vi "cam4 analyse.vi"() -> (0 "O8 chiffre":string, 1 "O7 chiffre":string, 2 "O1 chiffre":string, 3 "O2 chiffre":string, 4 "O5 chiffre":string, 5 "Y3 chiffre":string, 6 "Y6 chiffre":string, 7 "Y7 chiffre":string)   [LabVIEW 2019]
uses:
  <vilib>/vision/Classification.llb/IMAQ Classifier Read Options.ctl
  <vilib>/vision/NI_Vision_Development_Module.lvlib
panel:
  out "Coordinates":i32[](array[numeric])
  in  "Y7":T1={"Global Rectangle"=[0, 0, 1279, 959], "Contours"=[{"ID"=enum."External", "Type"=3, "Coordinates"=[0, 0, 1279, 959]}]} {"Contours"."Type" items=["No Selection", "Point", "Line", "Rectangle", "Oval", "Polygon", "Freehand Region", "Annulus", "Unused2", "Unused3", "Broken Line", "Freehand Line", "Rotated Rectangle"]}
  out "Y7":string[](array[string])
  in  "Y6":T1={"Global Rectangle"=[0, 0, 1279, 959], "Contours"=[{"ID"=enum."External", "Type"=3, "Coordinates"=[0, 0, 1279, 959]}]} {"Contours"."Type" items=["No Selection", "Point", "Line", "Rectangle", "Oval", "Polygon", "Freehand Region", "Annulus", "Unused2", "Unused3", "Broken Line", "Freehand Line", "Rotated Rectangle"]}
  out "Y6":string[](array[string])
  in  "Y3":T1={"Global Rectangle"=[0, 0, 1279, 959], "Contours"=[{"ID"=enum."External", "Type"=3, "Coordinates"=[0, 0, 1279, 959]}]} {"Contours"."Type" items=["No Selection", "Point", "Line", "Rectangle", "Oval", "Polygon", "Freehand Region", "Annulus", "Unused2", "Unused3", "Broken Line", "Freehand Line", "Rotated Rectangle"]}
  out "Y3":string[](array[string])
  in  "O1":T1={"Global Rectangle"=[0, 0, 1279, 959], "Contours"=[{"ID"=enum."External", "Type"=3, "Coordinates"=[0, 0, 1279, 959]}]} {"Contours"."Type" items=["No Selection", "Point", "Line", "Rectangle", "Oval", "Polygon", "Freehand Region", "Annulus", "Unused2", "Unused3", "Broken Line", "Freehand Line", "Rotated Rectangle"]}
  out "O1":string[](array[string])
  in  "O2":T1={"Global Rectangle"=[0, 0, 1279, 959], "Contours"=[{"ID"=enum."External", "Type"=3, "Coordinates"=[0, 0, 1279, 959]}]} {"Contours"."Type" items=["No Selection", "Point", "Line", "Rectangle", "Oval", "Polygon", "Freehand Region", "Annulus", "Unused2", "Unused3", "Broken Line", "Freehand Line", "Rotated Rectangle"]}
  out "O2":string[](array[string])
  in  "O5":T1={"Global Rectangle"=[0, 0, 1279, 959], "Contours"=[{"ID"=enum."External", "Type"=3, "Coordinates"=[0, 0, 1279, 959]}]} {"Contours"."Type" items=["No Selection", "Point", "Line", "Rectangle", "Oval", "Polygon", "Freehand Region", "Annulus", "Unused2", "Unused3", "Broken Line", "Freehand Line", "Rotated Rectangle"]}
  out "O5":string[](array[string])
  in  "O7":T1={"Global Rectangle"=[0, 0, 1279, 959], "Contours"=[{"ID"=enum."External", "Type"=3, "Coordinates"=[0, 0, 1279, 959]}]} {"Contours"."Type" items=["No Selection", "Point", "Line", "Rectangle", "Oval", "Polygon", "Freehand Region", "Annulus", "Unused2", "Unused3", "Broken Line", "Freehand Line", "Rotated Rectangle"]}
  out "O7":string[](array[string])
  in  "O8":T1={"Global Rectangle"=[640, 450, 686, 504], "Contours"=[{"ID"=enum."External", "Type"=3, "Coordinates"=[640, 450, 686, 504]}]} {"Contours"."Type" items=["No Selection", "Point", "Line", "Rectangle", "Oval", "Polygon", "Freehand Region", "Annulus", "Unused2", "Unused3", "Broken Line", "Freehand Line", "Rotated Rectangle"]}
  out "Image Out 2":T2(plugin-control)
  out "error out 2":errorcluster
  out "O8":string[](array[string])
  in  "error in":errorcluster
types:
  T1 = cluster{"Global Rectangle":i32[], "Contours":cluster{"ID":enum32{"External", "Internal"}, "Type":u32, "Coordinates":i32[]}[]}
  T2 = typedef "IMAQ Image.ctl" = refnum<image>
  T3 = typedef "IMAQ Classifier Read Options.ctl" = i32
  T4 = typedef "IMAQ Classifier Session.ctl" = refnum<k1>
  T5 = typedef "ROI Descriptor" = cluster{"Global Rectangle":i32[], "Contours":cluster{"ID":enum32{"External", "Internal"}, "Type":u32, "Coordinates":i32[]}[]}
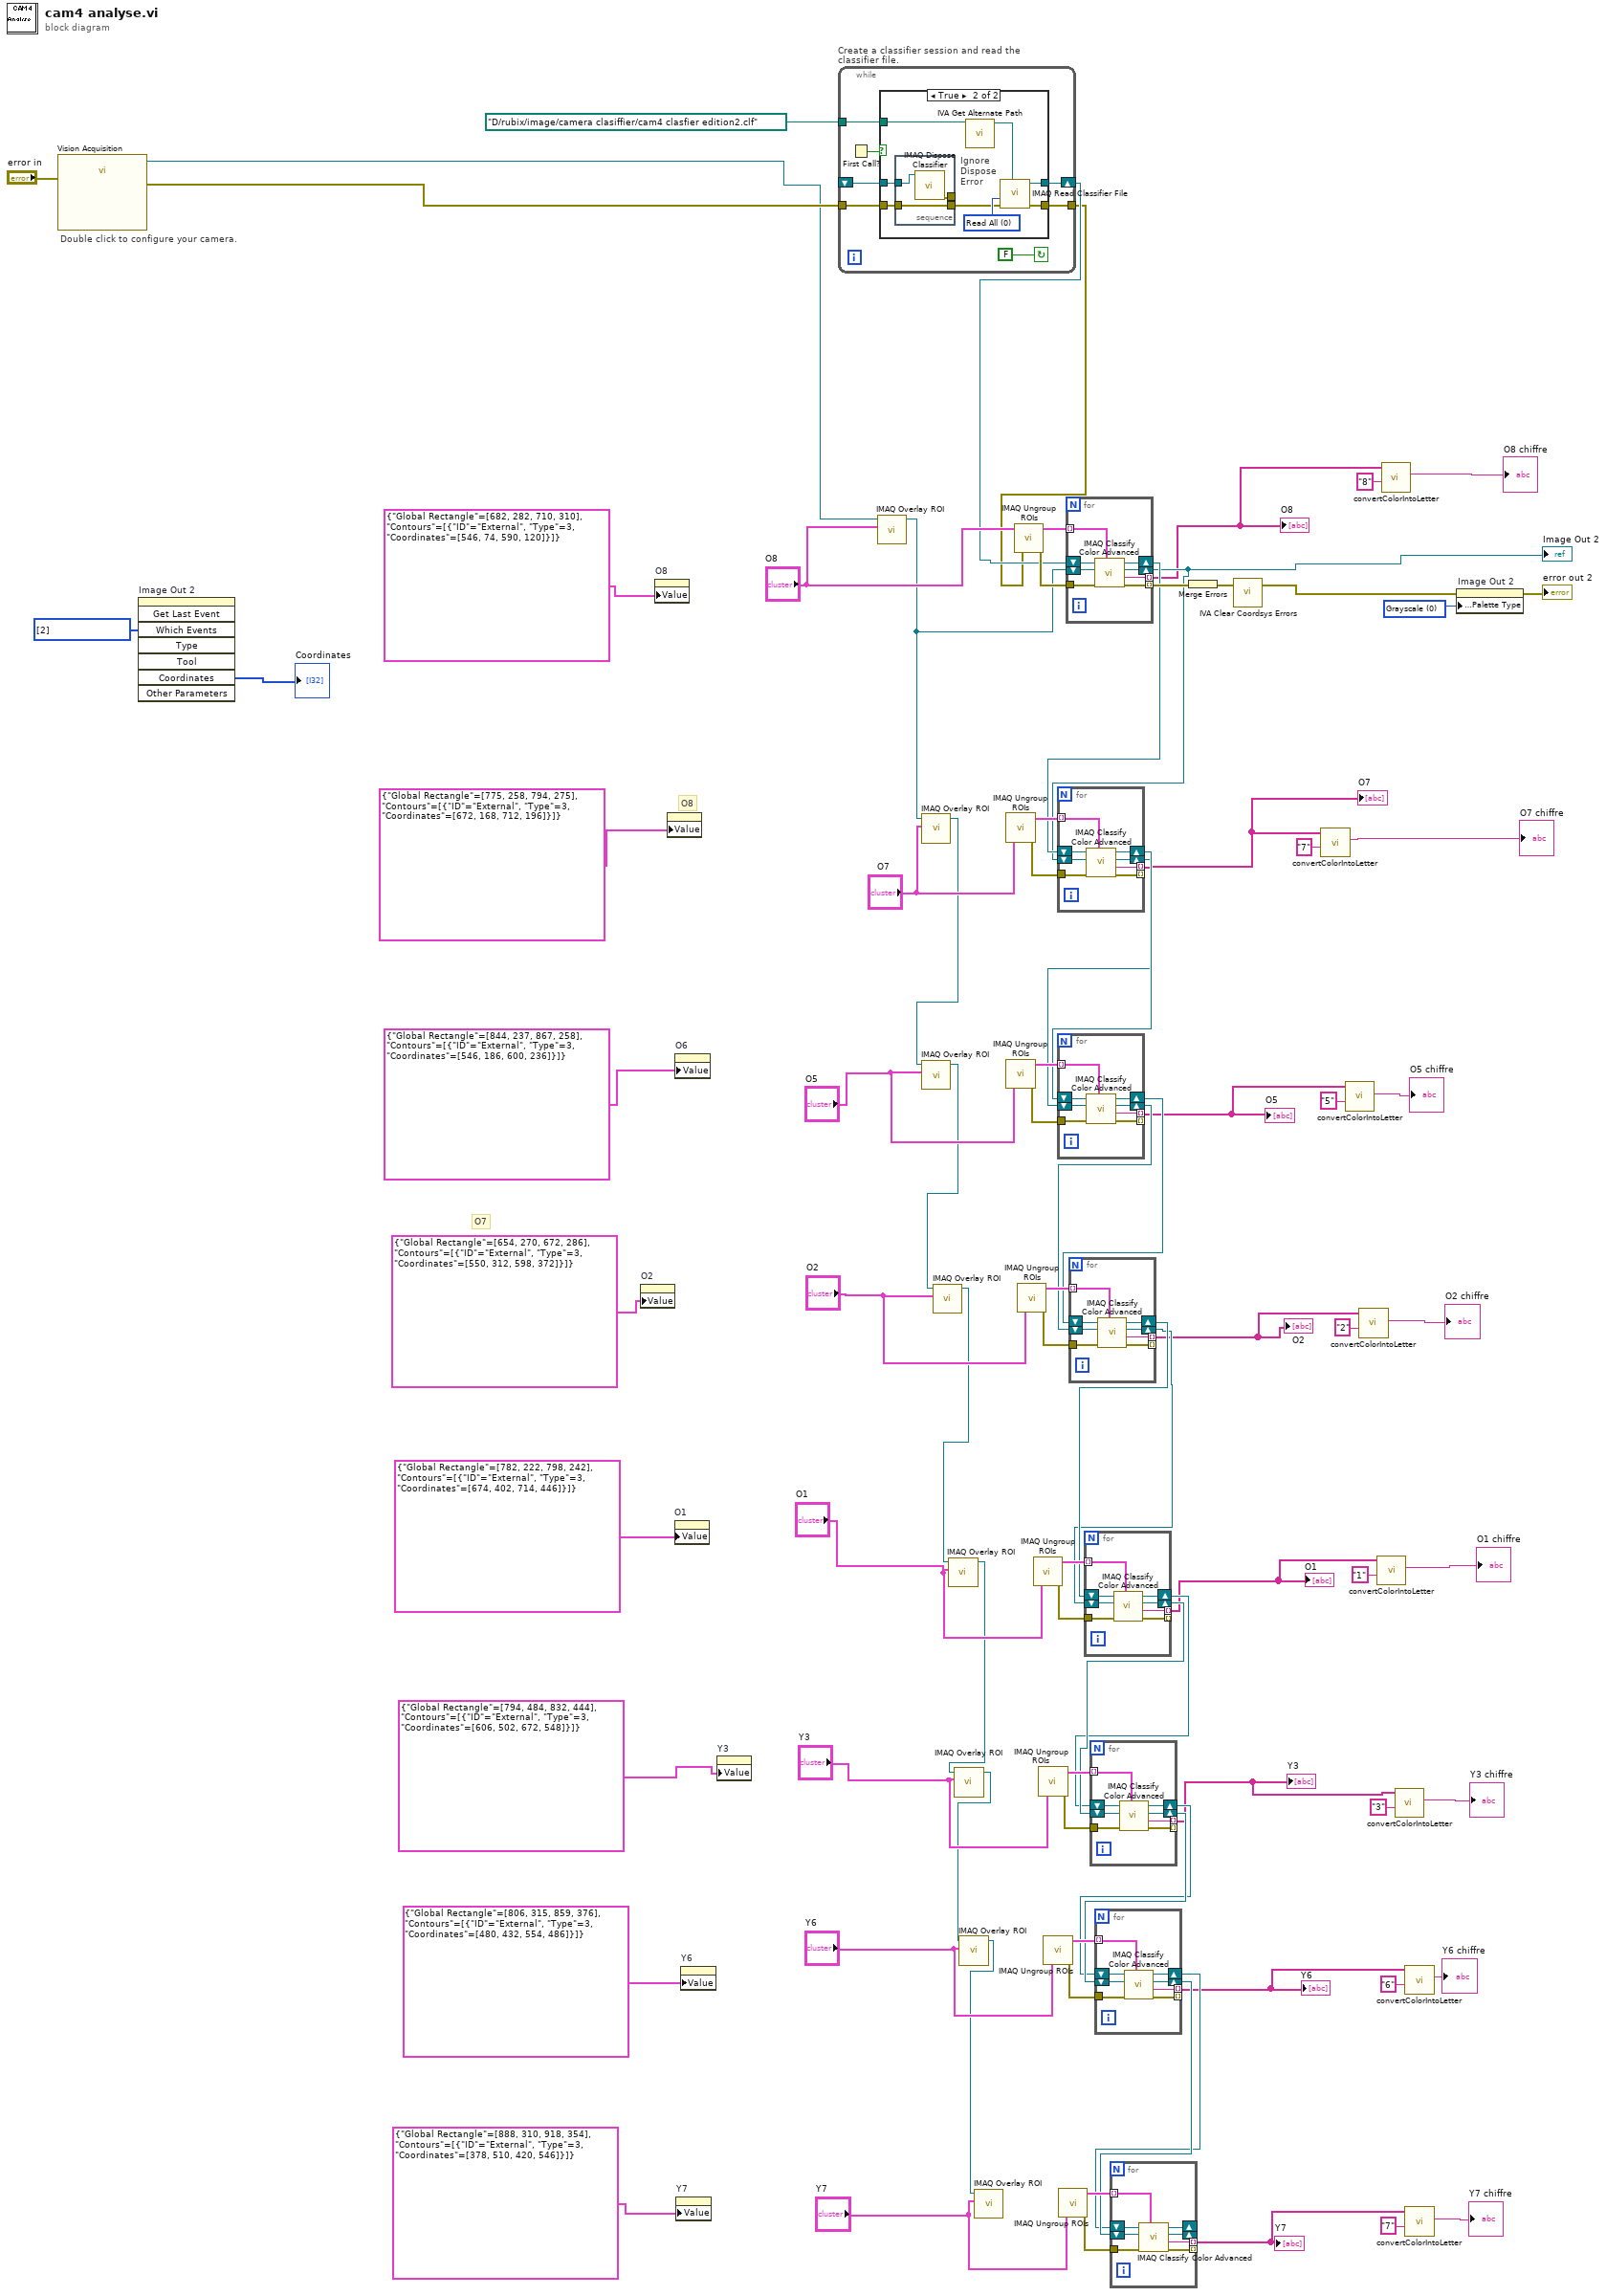
[diagram p0: block diagram]
diagram:
  w13 = i32[] [2] items=["No Event"=0, "Click Event"=1, "Draw Event"=2, "Size Event"=4, "Scroll Event"=5, "Double Click Event"=8] ("Which Events")
  w81 = u32 0 items=["Grayscale", "Binary", "Gradient", "Rainbow", "Temperature", "User Defined", "Binary 16 Bit", "Gradient 16 Bit", "Rainbow 16 Bit", "Temperature 16 Bit", "User Defined 16 Bit"] ("Palette Type")
  # "O8"
  # "O7"
  # "Double click to configure your camera."
  n1 = call "Vision Acquisition"("error in"="error in") -> ("Image Out"=w11:T2, "error out"=w89:errorcluster)  [unwired: 25 in]
  n2 = invoke on="Image Out 2" class="ImageControl" method="Get Last Event"("Which Events"=w13) -> ("Coordinates"=→"Coordinates":i32[])  [unwired: 7 in, 7 out]
  n3 = property on="O2" class="Clust (strict)"("Value"=T1 {"Global Rectangle"=[654, 270, 672, 286], "Contours"=[{"ID"=enum."External", "Type"=3, "Coordinates"=[550, 312, 598, 372]}]} ("ROI Descriptor (Color Classification 1)")) -> ()  [unwired: 2 in, 2 out]
  n4 = property on="O8" class="Clust (strict)"("Value"=T1 {"Global Rectangle"=[682, 282, 710, 310], "Contours"=[{"ID"=enum."External", "Type"=3, "Coordinates"=[546, 74, 590, 120]}]} ("ROI Descriptor (Color Classification 1)")) -> ()  [unwired: 2 in, 2 out]
  n5 = property class="Clust (strict)"("Value"=T1 {"Global Rectangle"=[775, 258, 794, 275], "Contours"=[{"ID"=enum."External", "Type"=3, "Coordinates"=[672, 168, 712, 196]}]} ("ROI Descriptor (Color Classification 1)")) -> ()  [unwired: 2 in, 2 out]
  n6 = property on="O1" class="Clust (strict)"("Value"=T1 {"Global Rectangle"=[782, 222, 798, 242], "Contours"=[{"ID"=enum."External", "Type"=3, "Coordinates"=[674, 402, 714, 446]}]} ("ROI Descriptor (Color Classification 1)")) -> ()  [unwired: 2 in, 2 out]
  n7 = property on="O6" class="Clust (strict)"("Value"=T1 {"Global Rectangle"=[844, 237, 867, 258], "Contours"=[{"ID"=enum."External", "Type"=3, "Coordinates"=[546, 186, 600, 236]}]} ("ROI Descriptor (Color Classification 1)")) -> ()  [unwired: 2 in, 2 out]
  n8 = property on="Y7" class="Clust (strict)"("Value"=T1 {"Global Rectangle"=[888, 310, 918, 354], "Contours"=[{"ID"=enum."External", "Type"=3, "Coordinates"=[378, 510, 420, 546]}]} ("ROI Descriptor (Color Classification 1)")) -> ()  [unwired: 2 in, 2 out]
  n9 = property on="Y6" class="Clust (strict)"("Value"=T1 {"Global Rectangle"=[806, 315, 859, 376], "Contours"=[{"ID"=enum."External", "Type"=3, "Coordinates"=[480, 432, 554, 486]}]} ("ROI Descriptor (Color Classification 1)")) -> ()  [unwired: 2 in, 2 out]
  n10 = property on="Y3" class="Clust (strict)"("Value"=T1 {"Global Rectangle"=[794, 484, 832, 444], "Contours"=[{"ID"=enum."External", "Type"=3, "Coordinates"=[606, 502, 672, 548]}]} ("ROI Descriptor (Color Classification 1)")) -> ()  [unwired: 2 in, 2 out]
  n11 = while "Create a classifier session and read the classifier file." {
    shift-right: [w97] -> w10
    shift-left: _ -> [w96]
    tunnel: w89 -> [w94]
    tunnel: [w93] -> w9
    tunnel: path "D:/rubix/image/camera clasiffier/cam4 clasfier edition2.clf" ("File Path") -> [w92]
    stop <- FALSE continue-if-true
    n12 = First Call?() -> (First Call?: T/F=w91:bool)
    n13 = case shown="True" w91 {
      tunnel: [w99 w106] -> w97
      tunnel: w96 -> [w99 w104]
      tunnel: w94 -> [w98 w103]
      tunnel: [w98 w105] -> w93
      tunnel: w92 -> [_ w101]
      frame False {
      }
      frame True {
        w107 = T3 0 items=["Read All", "Add Samples, Do Not Change Options", "Read Options, Do Not Add Samples"] ("Read Options")
        # "Ignore Dispose Error"
        n14 = stacked-sequence {
          tunnel: w104 -> [w110]
          tunnel: w103 -> [w109]
          tunnel: [w109] -> w102
          tunnel: [w108] -> _
          frame #0 {
            n15 = call "IMAQ Dispose Classifier"("Classifier Session"=w110) -> ("error out"=w108:errorcluster)  [unwired: 1 in, 9 out]
          }
        }
        n16 = call <vilib>:"IVA Get Alternate Path.vi"("Path In"=w101) -> ("Path Out"=w100:path)  [unwired: 10 out]
        n17 = call "IMAQ Read Classifier File"("File Path"=w100, "error in (no error)"=w102, "Read Options"=w107) -> ("error out"=w105:errorcluster, "Classifier Session"=w106:T4)  [unwired: 1 in, 6 out]
      }
    }
  }
  n18 = call "IMAQ Overlay ROI"("ROI Descriptor"="O8", "Image"=w11) -> ("Image Out"=w12:T2)  [unwired: 8 in, 1 out]
  n19 = call "IMAQ Overlay ROI"("ROI Descriptor"="O7", "Image"=w12) -> ("Image Out"=w74:T2)  [unwired: 8 in, 1 out]
  n20 = call "IMAQ Overlay ROI"("ROI Descriptor"="O5", "Image"=w74) -> ("Image Out"=w66:T2)  [unwired: 8 in, 1 out]
  n21 = call "IMAQ Overlay ROI"("ROI Descriptor"="O2", "Image"=w66) -> ("Image Out"=w58:T2)  [unwired: 8 in, 1 out]
  n22 = call "IMAQ Overlay ROI"("ROI Descriptor"="O1", "Image"=w58) -> ("Image Out"=w51:T2)  [unwired: 8 in, 1 out]
  n23 = call "IMAQ Overlay ROI"("ROI Descriptor"="Y3", "Image"=w51) -> ("Image Out"=w46:T2)  [unwired: 8 in, 1 out]
  n24 = call "IMAQ Overlay ROI"("ROI Descriptor"="Y6", "Image"=w46) -> ("Image Out"=w39:T2)  [unwired: 8 in, 1 out]
  n25 = call "IMAQ Overlay ROI"("ROI Descriptor"="Y7", "Image"=w39) -> ()  [unwired: 8 in, 2 out]
  n26 = call "IMAQ Ungroup ROIs"("ROI Descriptor"="O7") -> ("error out"=w80:errorcluster, "ROI Descriptors out"=w79:T5[])  [unwired: 1 in, 2 out]
  n27 = call "IMAQ Ungroup ROIs"("ROI Descriptor"="O5") -> ("error out"=w76:errorcluster, "ROI Descriptors out"=w75:T5[])  [unwired: 1 in, 2 out]
  n28 = call "IMAQ Ungroup ROIs"("error in (no error)"=w9, "ROI Descriptor"="O8") -> ("error out"=w87:errorcluster, "ROI Descriptors out"=w86:T5[])  [unwired: 2 out]
  n29 = call "IMAQ Ungroup ROIs"("ROI Descriptor"="O2") -> ("error out"=w69:errorcluster, "ROI Descriptors out"=w68:T5[])  [unwired: 1 in, 2 out]
  n30 = call "IMAQ Ungroup ROIs"("ROI Descriptor"="O1") -> ("error out"=w62:errorcluster, "ROI Descriptors out"=w61:T5[])  [unwired: 1 in, 2 out]
  n31 = call "IMAQ Ungroup ROIs"("ROI Descriptor"="Y3") -> ("error out"=w55:errorcluster, "ROI Descriptors out"=w54:T5[])  [unwired: 1 in, 2 out]
  n32 = call "IMAQ Ungroup ROIs"("ROI Descriptor"="Y6") -> ("error out"=w49:errorcluster, "ROI Descriptors out"=w48:T5[])  [unwired: 1 in, 2 out]
  n33 = call "IMAQ Ungroup ROIs"("ROI Descriptor"="Y7") -> ("error out"=w42:errorcluster, "ROI Descriptors out"=w41:T5[])  [unwired: 1 in, 2 out]
  n34 = for {
    tunnel: [w118] -> w19 mode=indexing
    tunnel: [w117] -> w85 mode=indexing
    tunnel: w87 -> [w115]
    tunnel: w86 -> [w114] mode=indexing
    shift-right: [w112] -> w21
    shift-left: w12 -> [w113]
    shift-right: [w111] -> w22
    shift-left: w10 -> [w116]
    n35 = call "IMAQ Classify Color Advanced"("ROI Descriptor"=w114, "error in (no error)"=w115, "Image"=w113, "Classifier Session"=w116) -> ("error out"=w117:errorcluster, "Class"=w118:string, "Image (dup)"=w112:T2, "Classifier Session (dup)"=w111:T4)  [unwired: 4 out]
  }
  "O8" <- w19
  "Image Out 2" <- w21
  n36 = for {
    tunnel: [w126] -> w16 mode=indexing
    tunnel: [w125] -> _ mode=indexing
    tunnel: w80 -> [w123]
    tunnel: w79 -> [w122] mode=indexing
    shift-right: [w120] -> w72
    shift-left: w21 -> [w121]
    shift-right: [w119] -> w73
    shift-left: w22 -> [w124]
    n37 = call "IMAQ Classify Color Advanced"("ROI Descriptor"=w122, "error in (no error)"=w123, "Image"=w121, "Classifier Session"=w124) -> ("error out"=w125:errorcluster, "Class"=w126:string, "Image (dup)"=w120:T2, "Classifier Session (dup)"=w119:T4)  [unwired: 4 out]
  }
  "O7" <- w16
  n38 = for {
    tunnel: [w134] -> w34 mode=indexing
    tunnel: [w133] -> _ mode=indexing
    tunnel: w76 -> [w131]
    tunnel: w75 -> [w130] mode=indexing
    shift-right: [w128] -> w65
    shift-left: w72 -> [w129]
    shift-right: [w127] -> w64
    shift-left: w73 -> [w132]
    n39 = call "IMAQ Classify Color Advanced"("ROI Descriptor"=w130, "error in (no error)"=w131, "Image"=w129, "Classifier Session"=w132) -> ("error out"=w133:errorcluster, "Class"=w134:string, "Image (dup)"=w128:T2, "Classifier Session (dup)"=w127:T4)  [unwired: 4 out]
  }
  "O5" <- w34
  n40 = for {
    tunnel: [w142] -> w33 mode=indexing
    tunnel: [w141] -> _ mode=indexing
    tunnel: w69 -> [w139]
    tunnel: w68 -> [w138] mode=indexing
    shift-right: [w136] -> w59
    shift-left: w65 -> [w137]
    shift-right: [w135] -> w60
    shift-left: w64 -> [w140]
    n41 = call "IMAQ Classify Color Advanced"("ROI Descriptor"=w138, "error in (no error)"=w139, "Image"=w137, "Classifier Session"=w140) -> ("error out"=w141:errorcluster, "Class"=w142:string, "Image (dup)"=w136:T2, "Classifier Session (dup)"=w135:T4)  [unwired: 4 out]
  }
  "O2" <- w33
  n42 = for {
    tunnel: [w150] -> w32 mode=indexing
    tunnel: [w149] -> _ mode=indexing
    tunnel: w62 -> [w147]
    tunnel: w61 -> [w146] mode=indexing
    shift-right: [w144] -> w53
    shift-left: w59 -> [w145]
    shift-right: [w143] -> w52
    shift-left: w60 -> [w148]
    n43 = call "IMAQ Classify Color Advanced"("ROI Descriptor"=w146, "error in (no error)"=w147, "Image"=w145, "Classifier Session"=w148) -> ("error out"=w149:errorcluster, "Class"=w150:string, "Image (dup)"=w144:T2, "Classifier Session (dup)"=w143:T4)  [unwired: 4 out]
  }
  "O1" <- w32
  n44 = for {
    tunnel: [w158] -> w31 mode=indexing
    tunnel: [w157] -> _ mode=indexing
    tunnel: w55 -> [w155]
    tunnel: w54 -> [w154] mode=indexing
    shift-right: [w152] -> w45
    shift-left: w53 -> [w153]
    shift-right: [w151] -> w44
    shift-left: w52 -> [w156]
    n45 = call "IMAQ Classify Color Advanced"("ROI Descriptor"=w154, "error in (no error)"=w155, "Image"=w153, "Classifier Session"=w156) -> ("error out"=w157:errorcluster, "Class"=w158:string, "Image (dup)"=w152:T2, "Classifier Session (dup)"=w151:T4)  [unwired: 4 out]
  }
  "Y3" <- w31
  n46 = for {
    tunnel: [w166] -> w30 mode=indexing
    tunnel: [w165] -> _ mode=indexing
    tunnel: w49 -> [w163]
    tunnel: w48 -> [w162] mode=indexing
    shift-right: [w160] -> w38
    shift-left: w45 -> [w161]
    shift-right: [w159] -> w37
    shift-left: w44 -> [w164]
    n47 = call "IMAQ Classify Color Advanced"("ROI Descriptor"=w162, "error in (no error)"=w163, "Image"=w161, "Classifier Session"=w164) -> ("error out"=w165:errorcluster, "Class"=w166:string, "Image (dup)"=w160:T2, "Classifier Session (dup)"=w159:T4)  [unwired: 4 out]
  }
  "Y6" <- w30
  n48 = for {
    tunnel: [w174] -> w29 mode=indexing
    tunnel: [w173] -> _ mode=indexing
    tunnel: w42 -> [w171]
    tunnel: w41 -> [w170] mode=indexing
    shift-right: [w168] -> _
    shift-left: w38 -> [w169]
    shift-right: [w167] -> _
    shift-left: w37 -> [w172]
    n49 = call "IMAQ Classify Color Advanced"("ROI Descriptor"=w170, "error in (no error)"=w171, "Image"=w169, "Classifier Session"=w172) -> ("error out"=w173:errorcluster, "Class"=w174:string, "Image (dup)"=w168:T2, "Classifier Session (dup)"=w167:T4)  [unwired: 4 out]
  }
  "Y7" <- w29
  n50 = Merge Errors(w85) -> (w84:errorcluster)
  n51 = call <vilib>:"IVA Clear Coordsys Errors.vi"("error in (no error)"=w84) -> ("error out"=w83:errorcluster)  [unwired: 10 in]
  n52 = call "convertColorIntoLetter.vi"("number"="7", "Array"=w16) -> ("String"=→"O7 chiffre":string)  [unwired: 9 in]
  n53 = call "convertColorIntoLetter.vi"("number"="5", "Array"=w34) -> ("String"=→"O5 chiffre":string)  [unwired: 9 in]
  n54 = call "convertColorIntoLetter.vi"("number"="2", "Array"=w33) -> ("String"=→"O2 chiffre":string)  [unwired: 9 in]
  n55 = call "convertColorIntoLetter.vi"("number"="1", "Array"=w32) -> ("String"=→"O1 chiffre":string)  [unwired: 9 in]
  n56 = call "convertColorIntoLetter.vi"("number"="8", "Array"=w19) -> ("String"=→"O8 chiffre":string)  [unwired: 9 in]
  n57 = call "convertColorIntoLetter.vi"("number"="3", "Array"=w31) -> ("String"=→"Y3 chiffre":string)  [unwired: 9 in]
  n58 = call "convertColorIntoLetter.vi"("number"="6", "Array"=w30) -> ("String"=→"Y6 chiffre":string)  [unwired: 9 in]
  n59 = call "convertColorIntoLetter.vi"("number"="7", "Array"=w29) -> ("String"=→"Y7 chiffre":string)  [unwired: 9 in]
  n60 = property on="Image Out 2" class="ImageControl"(error in=w83, "Palette:Palette Type"=w81) -> (error out=→"error out 2":errorcluster)  [unwired: 1 in, 1 out]
